vi "Start Logging.vi"(8 "Error In":errorcluster, 11 "Sinks":refnum<class "Log Sinks.lvclass">[](array[class])) -> (0 "Error Out":errorcluster, 3 "Logger":refnum<class "Log.lvclass">)   [LabVIEW 2019, in "TSC Event Logger.lvlib" / "Log.lvclass"]
doc: "Start logging events.\n\n<b>Code Developed By:</b>\nTechnology Service Corporation\nBloomington, IN 47403\nwww.tsc.com/atcs\n\nDeveloper:\nDaniel Coons"
uses:
  Log.lvclass
  Log Sinks/Log Sinks.lvclass
  Log Sinks/Log Sinks.lvclass/Log Sinks.ctl
  Log.lvclass/Log.ctl
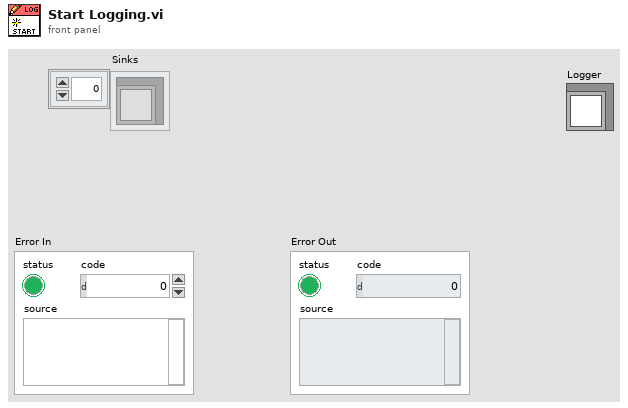
[diagram p1: front panel]
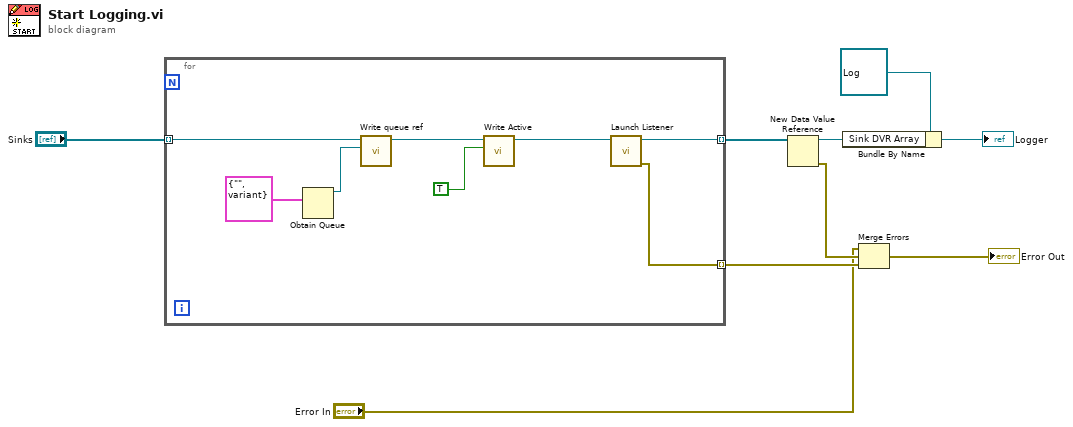
[diagram p0: block diagram]
diagram:
  n1 = for {
    tunnel: [w10] -> w9 mode=indexing
    tunnel: [w11] -> w4 mode=indexing
    tunnel: "Sinks" -> [w16] mode=indexing
    n2 = Obtain Queue(element data type=cluster{"msg":string, "data":variant} {"msg"="", "data"=variant}) -> (queue out=w14:refnum<queue>)  [unwired: 4 in, 2 out]
    n3 = call "Write queue ref.vi"("queue ref"=w14, "Log Sinks in"=w16) -> ("Log Sinks out"=w15:refnum<class "Log Sinks.lvclass">)  [unwired: 9 in]
    n4 = call "Write Active.vi"("Active?"=TRUE, "Log Sinks in"=w15) -> ("Log Sinks out"=w12:refnum<class "Log Sinks.lvclass">)  [unwired: 9 in]
    n5 = call "Launch Listener.vi"("Log Sinks in"=w12) -> ("error out"=w10:errorcluster, "Log Sinks out"=w11:refnum<class "Log Sinks.lvclass">)  [unwired: 9 in]
  }
  n6 = New Data Value Reference(data value=w4) -> (data value reference=w3:refnum<data-value>, error out=w2:errorcluster)  [unwired: 1 in]
  n7 = Bundle By Name(cluster=refnum<class "Log.lvclass"> refnum ("TSC Event Logger.lvlib:Log.lvclass"), "Sink DVR Array"=w3) -> (→"Logger":refnum<class "Log.lvclass">)
  n8 = Merge Errors("Error In", w2, w9) -> (→"Error Out":errorcluster)
